vi "Fit one AOI.vi"(0 "Image In":T3, 1 "derivative":T1(ring), 2 "fit type":u16, 5 "Image Type":u32, 7 "AOI (l, t, r, b)":u16[](array[numeric]), 9 "Data ID":string, 11 "error in":errorcluster, 12 "Guessed":T2(array[cluster]) {"Value" format="%.2f"}, 13 "max iterations":i32=200) -> (4 "Image Out":T3, 6 "Cancelled?":bool, 8 "integral":i32, 10 "Fit":T2(array[cluster]) {"Value" format="%.2f"}, 14 "mse":dbl format="%.4e", 15 "error out":errorcluster)   [LabVIEW 2016]
doc: "Calculates the parameter values that give the best fit between an analytical function and an experimentally determined image area of interest."
uses:
  <vilib>/vision/Image Controls.llb/IMAQ Image.ctl
  GLIMPSE Globals.vi
panel:
  out "Displayed fit is for":string
  in  "Do All":bool
  in  "Do 1":bool
  in  "Cancel":bool
  out "Input AOI":i16[][](graph)
  out "Fit":dbl[][](graph)
  out "Residual":dbl[][](graph)
  # "Parameters that are not used interactively"
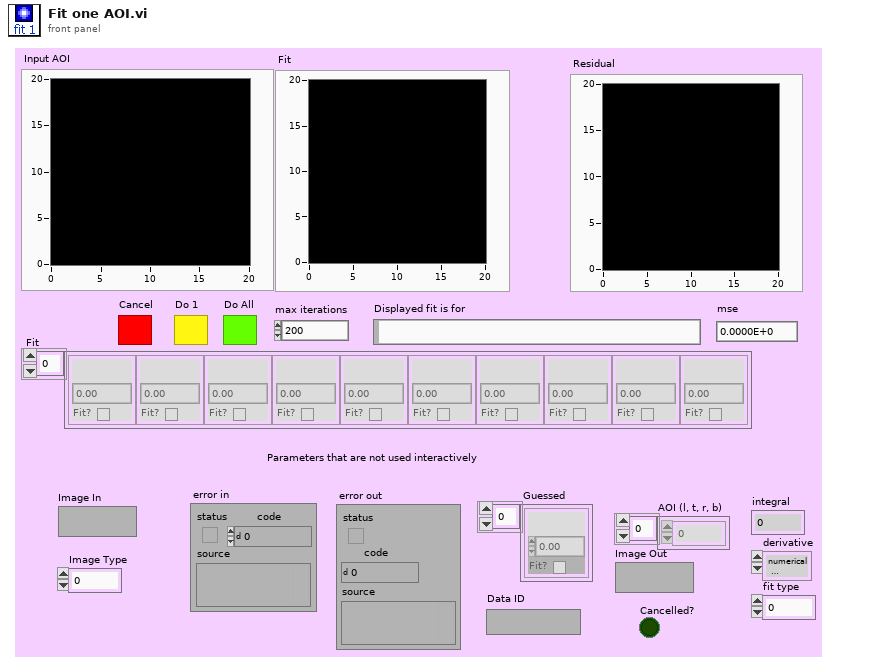
[diagram p1: front panel]
types:
  T1 = enum32{"numerical calculation", "formula calculation"}
  T2 = cluster{"Name":string, "Value":dbl, "Fit?":bool}[]
  T3 = typedef "IMAQ Image.ctl" = refnum<image>
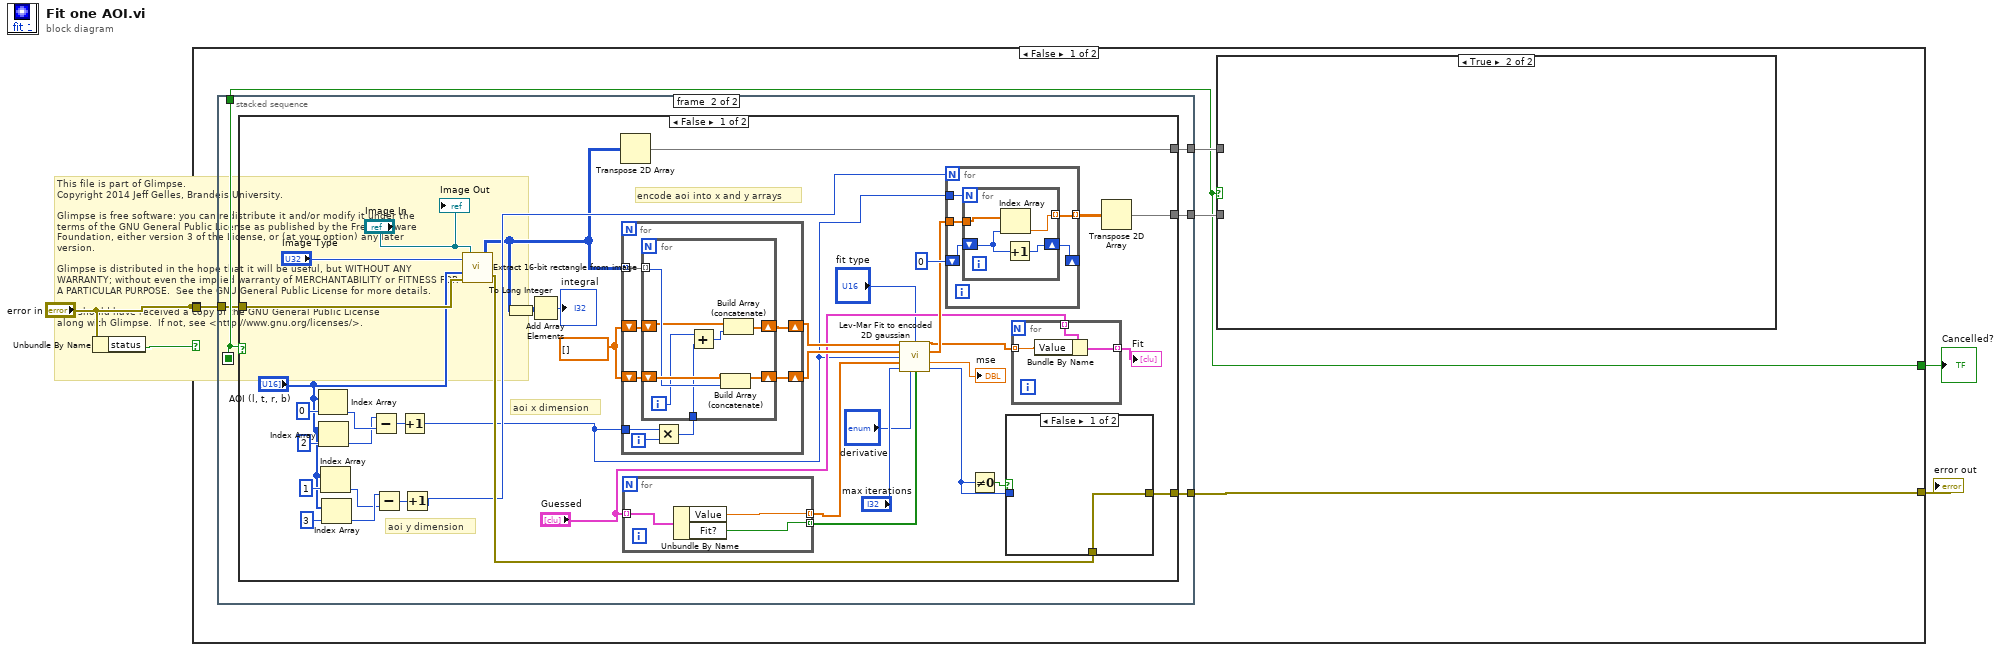
[diagram p0: block diagram]
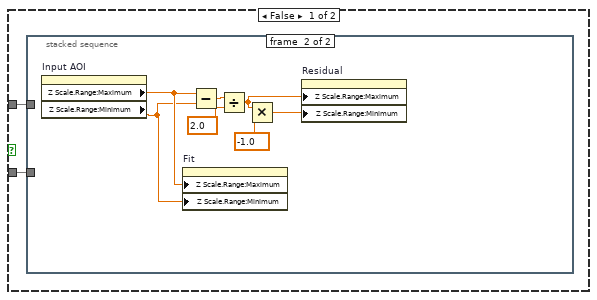
[diagram p2: hidden frame]
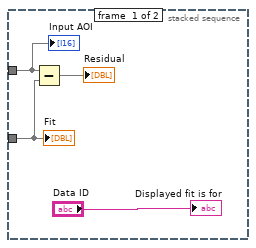
[diagram p3: hidden frame]
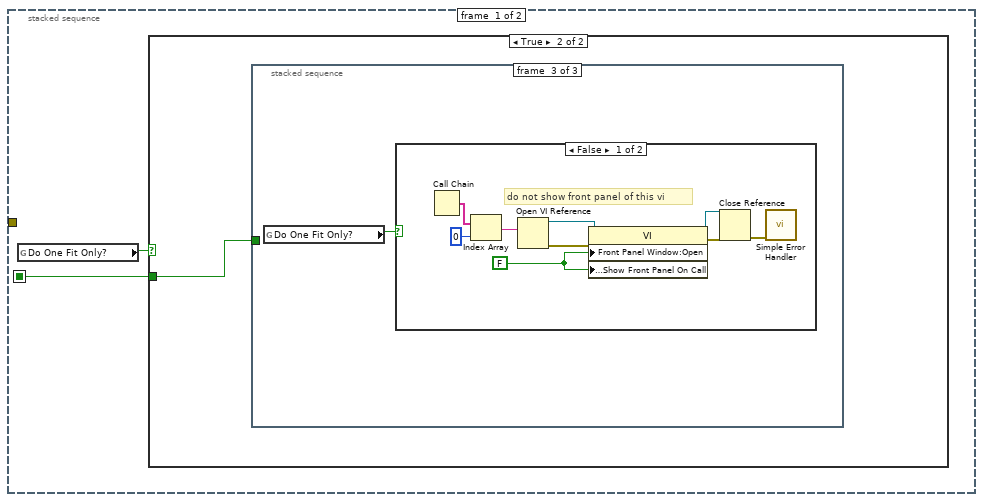
[diagram p4: hidden frame]
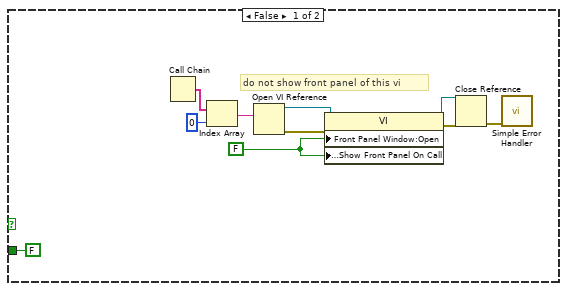
[diagram p5: hidden frame]
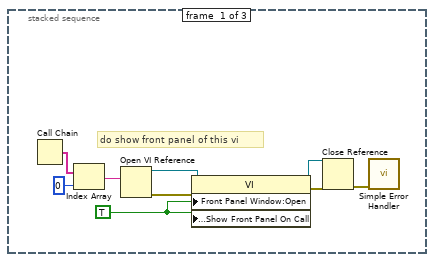
[diagram p6: hidden frame]
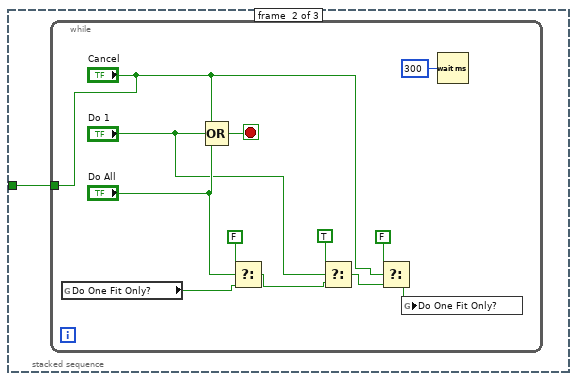
[diagram p7: hidden frame]
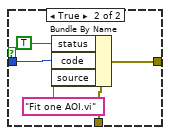
[diagram p9: hidden frame]
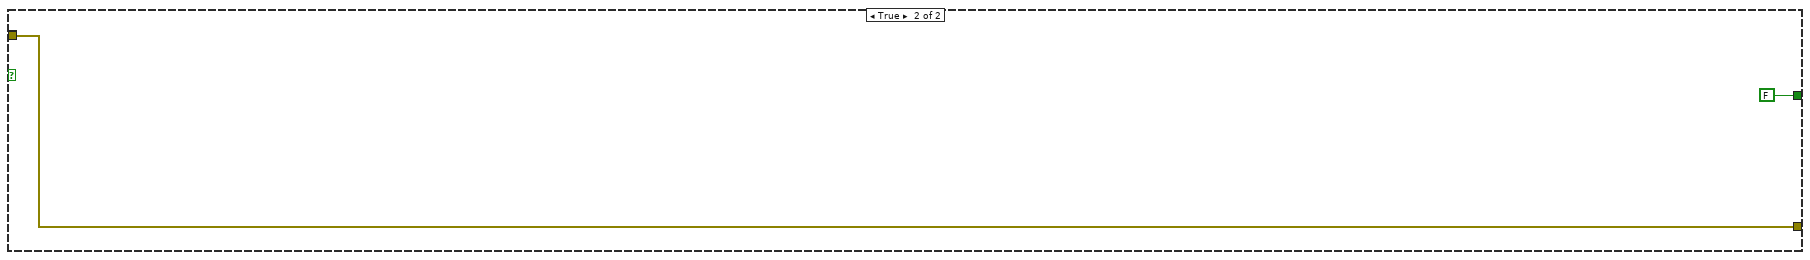
[diagram p11: hidden frame]
diagram:
  # "This file is part of Glimpse. \nCopyright 2014 Jeff Gelles, Brandeis University.    \n\nGlimpse is free software: you can redistribute it and/or modify it under the \nterms of the GNU General Public License as published by the Free Software \nFoundation, either version 3 of the License, or (at your option) any later \nversion.\n\nGlimpse is distributed in the hope that it will be useful, but WITHOUT ANY \nWARRANTY; without even the implied warranty of MERCHANTABILITY or FITNESS FOR \nA PARTICULAR PURPOSE.  See the GNU General Public License for more details.\n\nYou should have received a copy of the GNU General Public License\nalong with Glimpse.  If not, see <http://www.gnu.org/licenses/>."
  n1 = Unbundle By Name("error in") -> ("status"=w3:bool)
  n2 = case shown="False" w3 {
    tunnel: "error in" -> [w7 _]
    tunnel: [w6 w152] -> w4
    tunnel: "error in" -> [_ w152]
    tunnel: [w5 FALSE ("Cancel")] -> w1
    frame False {
      n3 = stacked-sequence {
        seq-local: [w24 _] -> [_ w70]
        tunnel: [_ w72] -> w9
        tunnel: [_ w71] -> w8
        tunnel: [_ w70] -> w5
        tunnel: w7 -> [_ w69]
        tunnel: [_ w68] -> w6
        frame #0 {
          n4 = global read "GLIMPSE Globals.vi" "Do One Fit Only?"() -> (w23:bool)
          n5 = case shown="True" w23 {
            tunnel: [FALSE ("Cancel") w35] -> w24
            frame False {
              w25 = FALSE ("Front Panel Window:Open")
              # "do not show front panel of this vi"
              n6 = Call Chain() -> (call chain=w33:string[])
              n7 = Index Array(array=w33, index=0 ("Index")) -> (element=w31:string)
              n8 = Open VI Reference(vi path=w31) -> (vi reference=w30:refnum<vi>, error out=w29:errorcluster)  [unwired: 1 in, 4 out]
              n9 = property class="VI"(reference=w30, error in=w29, "Front Panel Window:Open"=w25, "Execution:Show Front Panel On Call"=w25) -> (reference out=w28:refnum<vi>, error out=w27:errorcluster)
              n10 = Close Reference(reference=w28, error in (no error)=w27) -> (error out=w26:errorcluster)
              n11 = call <vilib>:"Simple Error Handler.vi"("error in (no error)"=w26) -> ()  [unwired: 1 in, 8 out]
            }
            frame True {
              n12 = stacked-sequence {
                tunnel: [_ w45 _] -> w35
                frame #0 {
                  w36 = TRUE ("Front Panel Window:Open")
                  # "do show front panel of this vi"
                  n13 = Call Chain() -> (call chain=w44:string[])
                  n14 = Index Array(array=w44, index=0 ("Index")) -> (element=w42:string)
                  n15 = Open VI Reference(vi path=w42) -> (vi reference=w41:refnum<vi>, error out=w40:errorcluster)  [unwired: 1 in, 4 out]
                  n16 = property class="VI"(reference=w41, error in=w40, "Front Panel Window:Open"=w36, "Execution:Show Front Panel On Call"=w36) -> (reference out=w39:refnum<vi>, error out=w38:errorcluster)
                  n17 = Close Reference(reference=w39, error in (no error)=w38) -> (error out=w37:errorcluster)
                  n18 = call <vilib>:"Simple Error Handler.vi"("error in (no error)"=w37) -> ()  [unwired: 1 in, 8 out]
                }
                frame #1 {
                  n19 = while {
                    tunnel: ["Cancel"] -> w45
                    stop <- w57 stop-if-true
                    n20 = global read "GLIMPSE Globals.vi" "Do One Fit Only?"() -> (w54:bool)
                    n21 = Compound Arithmetic op=OR("Cancel", "Do 1", "Do All") -> (w57:bool)
                    n22 = Select(t=FALSE, s="Do All", f=w54) -> (s? t:f=w53:bool)
                    n23 = Select(t=TRUE, s="Do 1", f=w53) -> (s? t:f=w48:bool)
                    n24 = Select(t=FALSE, s="Cancel", f=w48) -> (s? t:f=w46:bool)
                    n25 = global write "GLIMPSE Globals.vi" "Do One Fit Only?"(w46) -> ()
                    n26 = Wait (ms)(milliseconds to wait=u32 300) -> ()  [unwired: 1 out]
                  }
                }
                frame #2 {
                  n27 = global read "GLIMPSE Globals.vi" "Do One Fit Only?"() -> (w58:bool)
                  n28 = case shown="False" w58 {
                    frame False {
                      w59 = FALSE ("Front Panel Window:Open")
                      # "do not show front panel of this vi"
                      n29 = Call Chain() -> (call chain=w67:string[])
                      n30 = Index Array(array=w67, index=0 ("Index")) -> (element=w65:string)
                      n31 = Open VI Reference(vi path=w65) -> (vi reference=w64:refnum<vi>, error out=w63:errorcluster)  [unwired: 1 in, 4 out]
                      n32 = property class="VI"(reference=w64, error in=w63, "Front Panel Window:Open"=w59, "Execution:Show Front Panel On Call"=w59) -> (reference out=w62:refnum<vi>, error out=w61:errorcluster)
                      n33 = Close Reference(reference=w62, error in (no error)=w61) -> (error out=w60:errorcluster)
                      n34 = call <vilib>:"Simple Error Handler.vi"("error in (no error)"=w60) -> ()  [unwired: 1 in, 8 out]
                    }
                    frame True {
                    }
                  }
                }
              }
            }
          }
        }
        frame #1 {
          n35 = case shown="False" w70 {
            tunnel: [w111 _] -> w72
            tunnel: [w110 _] -> w71
            tunnel: w69 -> [w95 w150]
            tunnel: [w91 w150] -> w68
            frame False {
              w105 = dbl[] []
              # "aoi y dimension"
              # "aoi x dimension"
              # "encode aoi into x and y arrays"
              n36 = Index Array(array="AOI (l, t, r, b)", index=0) -> (element=w97:u16)
              n37 = Index Array(array="AOI (l, t, r, b)", index=2) -> (element=w96:u16)
              n38 = Index Array(array="AOI (l, t, r, b)", index=1) -> (element=w85:u16)
              n39 = Index Array(array="AOI (l, t, r, b)", index=3) -> (element=w86:u16)
              n40 = Subtract(x=w96, y=w97) -> (x-y=w98:u16)
              n41 = Subtract(x=w86, y=w85) -> (x-y=w84:u16)
              n42 = Increment(x=w98) -> (x+1=w79:u16)
              n43 = Increment(x=w84) -> (x+1=w80:u16)
              n44 = call "Extract 16-bit rectangle from image.vi"("error in"=w95, "AOI (t, l, b, r)"="AOI (l, t, r, b)", "Image pixel depth"="Image Type", "Image in"="Image In") -> ("error out"=w93:errorcluster, "Image Pixels (I16)"=w75:i16[][])
              n45 = To Long Integer(number=w75) -> (32bit integer=w73:i32[][])
              n46 = Add Array Elements(numeric array=w73) -> (sum=→"integral":i32)
              n47 = Transpose 2D Array(2D array=w75) -> (transposed array=w110:i16[][])
              n48 = for {
                tunnel: w75 -> [w132] mode=indexing
                shift-right: [w131] -> w104
                shift-left: w105 -> [w128]
                shift-right: [w130] -> w103
                shift-left: w105 -> [w129]
                tunnel: w79 -> [w127]
                i -> [w126]
                n49 = Multiply(x=w127, y=w126) -> (x*y=w125:i32)
                n50 = for {
                  tunnel: w132 -> [w138] mode=indexing
                  shift-right: [w140] -> w130
                  shift-left: w129 -> [w139]
                  shift-right: [w137] -> w131
                  shift-left: w128 -> [w136]
                  tunnel: w125 -> [w134]
                  i -> [w133]
                  n51 = Add(x=w133, y=w134) -> (x+y=w135:i32)
                  n52 = Build Array (concatenate)(w139, w138) -> (w140:dbl[])
                  n53 = Build Array (concatenate)(w136, w135) -> (w137:dbl[])
                }
              }
              n54 = for {
                tunnel: "Guessed" -> [w118] mode=indexing
                tunnel: [w117] -> w90 mode=indexing
                tunnel: [w116] -> w78 mode=indexing
                n55 = Unbundle By Name(w118) -> ("Value"=w117:dbl, "Fit?"=w116:bool)
              }
              n56 = call "Lev-Mar Fit to encoded 2D gaussian.vi"("X"=w104, "fit type"="fit type", "Y"=w103, "code"=w79, "Initial Guess Coefficients"=w90, "max iteration"="max iterations", "derivative"="derivative", "Fit this coeff?"=w78) -> ("Best Fit Coefficients"=w88:dbl[], "Best Fit"=w107:dbl[], "mse"=→"mse":dbl, "error"=w92:i32)  [unwired: 1 in, 3 out]
              n57 = for {
                N: w80 -> [_]
                tunnel: w107 -> [w145]
                tunnel: [w144] -> w109 mode=indexing
                shift-right: [w142] -> _
                shift-left: i16 0 -> [w143]
                tunnel: w79 -> [w141]
                n58 = for {
                  N: w141 -> [_]
                  tunnel: w145 -> [w148]
                  tunnel: [w149] -> w144 mode=indexing
                  shift-right: [w147] -> w142
                  shift-left: w143 -> [w146]
                  n59 = Index Array(array=w148, index=w146) -> (element=w149:dbl)
                  n60 = Increment(x=w146) -> (x+1=w147:i16)
                }
              }
              n61 = Not Equal To 0?(x=w92) -> (x != 0?=w94:bool)
              n62 = case shown="False" w94 {
                tunnel: w93 -> [w119 w124]
                tunnel: w92 -> [_ w122]
                tunnel: [w119 w120] -> w91
                frame False {
                }
                frame True {
                  n63 = Bundle By Name(cluster=w124, "status"=TRUE, "code"=w122, "source"="Fit one AOI.vi") -> (w120:errorcluster)
                }
              }
              n64 = for {
                tunnel: "Guessed" -> [w115] mode=indexing
                tunnel: w88 -> [w114] mode=indexing
                tunnel: [w113] -> w87 mode=indexing
                n65 = Bundle By Name(cluster=w115, "Value"=w114) -> (w113:cluster{"Name":string, "Value":dbl, "Fit?":bool})
              }
              "Fit" <- w87
              n66 = Transpose 2D Array(2D array=w109) -> (transposed array=w111:dbl[][])
              "Image Out" <- "Image In"
            }
            frame True {
            }
          }
        }
      }
      n67 = case shown="True" w5 {
        tunnel: w9 -> [w11 _]
        tunnel: w8 -> [w10 _]
        frame False {
          n68 = stacked-sequence {
            tunnel: w11 -> [w15 _]
            tunnel: w10 -> [w13 _]
            frame #0 {
              n69 = Subtract(x=w13, y=w15) -> (x-y=→"Residual":dbl[][])
              "Fit" <- w15
              "Input AOI" <- w13
              "Displayed fit is for" <- "Data ID"
            }
            frame #1 {
              n70 = property on="Input AOI" class="IntGraph (strict)"() -> ("Z Scale.Range:Maximum"=w22:dbl, "Z Scale.Range:Minimum"=w21:dbl)  [unwired: 2 in, 2 out]
              n71 = property on="Fit" class="IntGraph (strict)"("Z Scale.Range:Maximum"=w22, "Z Scale.Range:Minimum"=w21) -> ()  [unwired: 2 in, 2 out]
              n72 = Subtract(x=w22, y=w21) -> (x-y=w20:dbl)
              n73 = Divide(x=w20, y=2.0) -> (x/y=w16:dbl)
              n74 = Multiply(x=w16, y=-1.0) -> (x*y=w17:dbl)
              n75 = property on="Residual" class="IntGraph (strict)"("Z Scale.Range:Maximum"=w16, "Z Scale.Range:Minimum"=w17) -> ()  [unwired: 2 in, 2 out]
            }
          }
        }
        frame True {
        }
      }
    }
    frame True {
    }
  }
  "error out" <- w4
  "Cancelled?" <- w1
